vi "Set Value.vi"(7 "TOML string":string, 8 "error in (no error)":errorcluster, 9 "start position":i32, 10 "Value":T3, 11 "Values in":T2[](array[typedef])) -> (0 "error out":errorcluster, 1 "offset past match":i32, 2 "State":T1, 3 "Values out":T2[](array[typedef]))   [LabVIEW 2015, in "JSON.lvlib"]
uses:
  JSON.lvlib
  Value.ctl
  Value Type.ctl
  Context.ctl
  State.ctl
  Object Context.ctl
  Name-Value Pair.ctl
  Array Context.ctl
  <vilib>/regexp/Match Regular Expression.xnode
panel:
  in  "Define":bool=TRUE
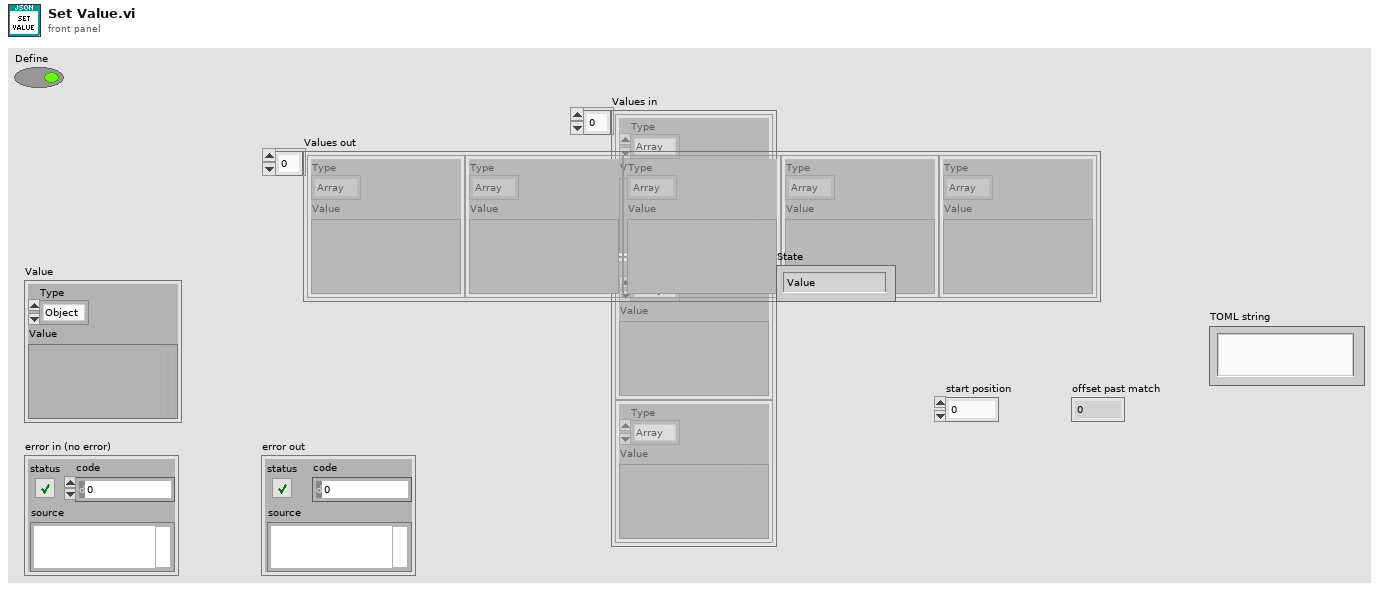
[diagram p1: front panel]
types:
  T1 = typedef "JSON.lvlib/State.ctl" = enum16{"Value", "Object"}
  T2 = typedef "JSON.lvlib/Context.ctl" = cluster{"Type":enum16{"Array", "Object", "Root"}, "Value":variant}
  T3 = typedef "JSON.lvlib/Value.ctl" = cluster{"Type":T4, "Value":variant}
  T4 = typedef "JSON.lvlib/Value Type.ctl" = enum16{"Object", "Array", "String", "Number", "Boolean", "Null"}
  T5 = typedef "JSON.lvlib/Object Context.ctl" = cluster{"Object":T6[], "Key":string}
  T6 = typedef "JSON.lvlib/Name-Value Pair.ctl" = cluster{"Name":string, "Value":T3}
  T7 = typedef "JSON.lvlib/Array Context.ctl" = cluster{"Array":T3[]}
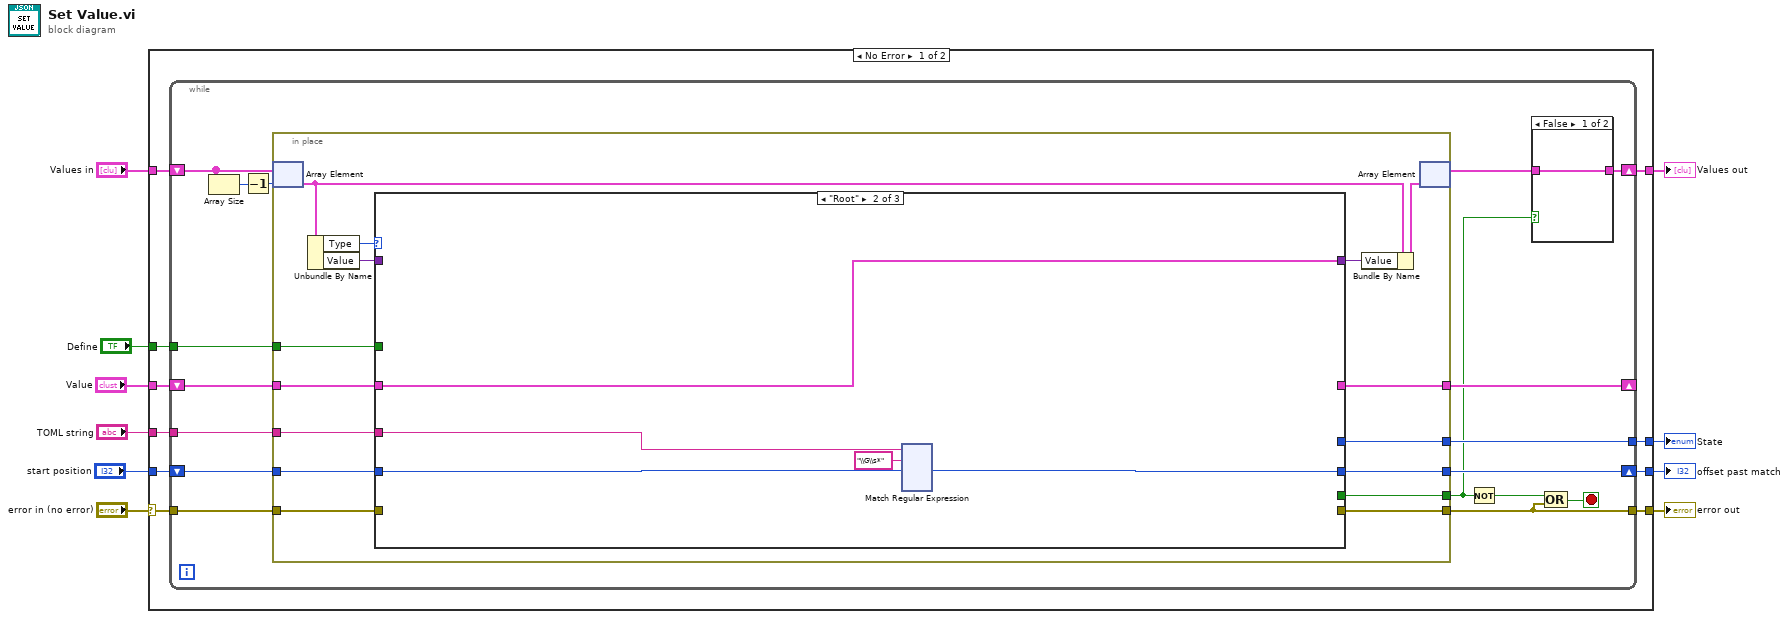
[diagram p0: block diagram]
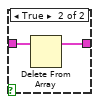
[diagram p2: hidden frame]
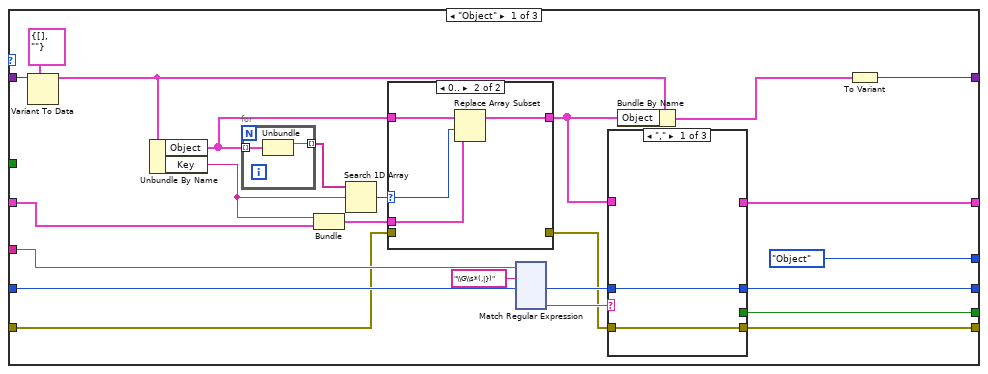
[diagram p3: hidden frame]
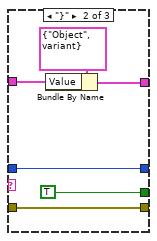
[diagram p4: hidden frame]
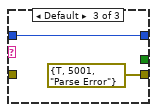
[diagram p5: hidden frame]
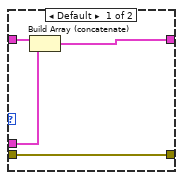
[diagram p6: hidden frame]
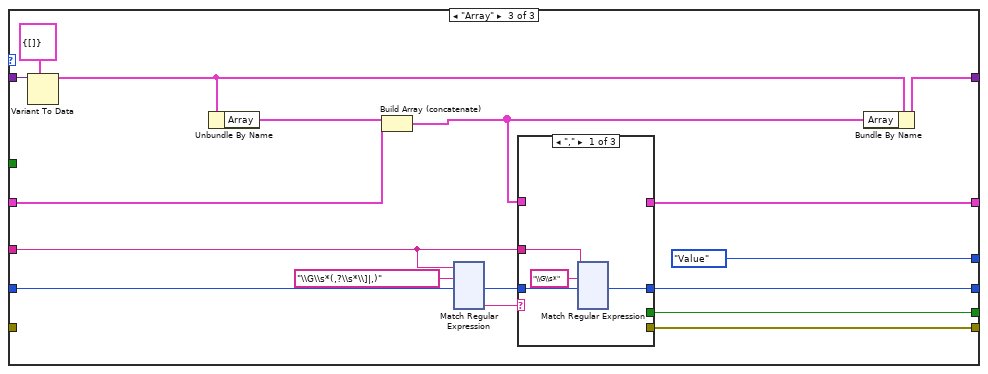
[diagram p7: hidden frame]
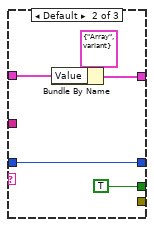
[diagram p8: hidden frame]
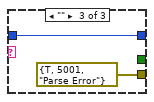
[diagram p9: hidden frame]
diagram:
  n1 = case shown="No Error" "error in (no error)" {
    selector: "error in (no error)" -> [w15 w599]
    tunnel: "Values in" -> [w20 w597]
    tunnel: [w19 w597] -> w9
    tunnel: "Value" -> [w18 _]
    tunnel: [w17 _] -> w7
    tunnel: [w16 w599] -> w6
    tunnel: "start position" -> [w14 w598]
    tunnel: "TOML string" -> [w13 _]
    tunnel: [w12 w598] -> w2
    tunnel: "Define" -> [w11 _]
    frame No Error {
      n2 = while {
        tunnel: [w33] -> w17
        tunnel: w13 -> [w28]
        shift-right: [w26] -> w12
        shift-left: w14 -> [w29]
        tunnel: w15 -> [w32]
        tunnel: [w30] -> w16
        shift-right: [w25] -> _
        shift-left: w18 -> [w34]
        shift-right: [w24] -> w19
        shift-left: w20 -> [w35]
        tunnel: w11 -> [w23]
        stop <- w31 stop-if-true
        n3 = Array Size(array=w35) -> (size(s)=w37:i32)
        n4 = Decrement(x=w37) -> (x-1=w36:i32)
        n5 = in-place {
          in-place-border: w34 -> [w50]
          in-place-border: [w49] -> w33
          in-place-border: [w48] -> w30
          in-place-border: w32 -> [w47]
          in-place-border: [w44] -> w21
          in-place-border: w29 -> [w46]
          in-place-border: w28 -> [w45]
          in-place-border: [w43] -> w25
          in-place-border: [w42] -> w26
          in-place-border: w23 -> [w41]
          n6 = in-place-array #1(w35, w36) -> (w53:T2)
          n7 = Unbundle By Name(w53) -> ("Type"=w55:enum16{"Array", "Object", "Root"}, "Value"=w54:variant)
          n8 = case shown="\"Root\"" w55 {
            tunnel: w54 -> [w79 _ w353]
            tunnel: w50 -> [w73 w220 w342]
            tunnel: [w58 w220 w352] -> w52
            tunnel: [State."Object" ("State") _ State."Value" ("State")] -> w49
            tunnel: [w60 _ w345] -> w48
            tunnel: w47 -> [w57 _ _]
            tunnel: w46 -> [w69 w217 w348]
            tunnel: w45 -> [w68 w218 w344]
            tunnel: [w64 _ w349] -> w44
            tunnel: [w62 _ w346] -> w43
            tunnel: [w61 w216 w347] -> w42
            tunnel: w41 -> [_ _ _]
            frame "Object" {
              n9 = Variant To Data(type=T5 {"Object"=[], "Key"=""} ("Table Context"), Variant=w79) -> (data=w72:T5)  [unwired: 1 in, 1 out]
              n10 = Unbundle By Name(w72) -> ("Object"=w75:T6[], "Key"=w74:string)
              n11 = for {
                tunnel: w75 -> [w215] mode=indexing
                tunnel: [w214] -> w77 mode=indexing
                n12 = Unbundle(w215) -> ("Name"=w214:string)  [unwired: 1 out]
              }
              n13 = Bundle("Key"=w74, "Value"=w73) -> (w71:cluster{"Key":string, "Value":T3})  [unwired: 1 in]
              n14 = Search 1D Array(1D array=w77, element=w74) -> (index of element=w76:i32)  [unwired: 1 in]
              n15 = case shown="0.." w76 {
                selector: w76 -> [_ w212]
                tunnel: w75 -> [w209 w213]
                tunnel: [w208 w210] -> w63
                tunnel: w71 -> [w207 w211]
                tunnel: w57 -> [w206 _]
                tunnel: [w206 _] -> w56
                frame Default {
                  n16 = Build Array (concatenate)(w209, w207) -> (w208:T6[])
                }
                frame 0.. {
                  n17 = Replace Array Subset(array=w213, new element=w211, index=w212) -> (w210:T6[])
                }
              }
              n18 = xnode "Match Regular Expression"("input string"=w68, "regular expression"="\\G\\s*(,|})", "offset (0)"=w69) -> ("offset past match"=w65:i32, "submatch 1"=w66:string)  [unwired: 3 in, 4 out]
              n19 = case shown="\",\"" w66 {
                tunnel: w65 -> [w197 w199 w205]
                tunnel: [_ TRUE _] -> w64
                tunnel: w63 -> [_ w201 _]
                tunnel: [_ w200 _] -> w62
                tunnel: [w197 w199 w205] -> w61
                tunnel: [w196 w198 errorcluster {"status"=TRUE, "code"=5001, "source"="Parse Error"} ("error constant")] -> w60
                tunnel: w56 -> [w196 w198 _]
                frame "," {
                }
                frame "}" {
                  n20 = Bundle By Name(cluster=T3 {"Type"=enum."Object", "Value"=variant} ("Value"), "Value"=w201) -> (w200:T3)
                }
                frame Default {
                }
              }
              n21 = Bundle By Name(cluster=w72, "Object"=w63) -> (w59:T5)
              n22 = To Variant(anything=w59) -> (Variant=w58:variant)
            }
            frame "Root" {
              n23 = xnode "Match Regular Expression"("input string"=w218, "regular expression"="\\G\\s*", "offset (0)"=w217) -> ("offset past match"=w216:i32)  [unwired: 3 in, 5 out]
            }
            frame "Array" {
              n24 = Variant To Data(type=T7 {"Array"=[]} ("Array Context"), Variant=w353) -> (data=w343:T7)  [unwired: 1 in, 1 out]
              n25 = Unbundle By Name(w343) -> ("Array"=w337:T3[])
              n26 = Build Array (concatenate)(w337, w342) -> (w338:T3[])
              n27 = xnode "Match Regular Expression"("input string"=w344, "regular expression"="\\G\\s*(,?\\s*\\]|,)", "offset (0)"=w348) -> ("offset past match"=w339:i32, "submatch 1"=w340:string)  [unwired: 3 in, 4 out]
              n28 = case shown="\",\"" w340 {
                tunnel: w339 -> [w471 w590 w596]
                tunnel: [_ TRUE _] -> w349
                tunnel: w338 -> [_ w592 _]
                tunnel: [_ w591 _] -> w346
                tunnel: [w470 w590 w596] -> w347
                tunnel: [_ _ errorcluster {"status"=TRUE, "code"=5001, "source"="Parse Error"} ("error constant")] -> w345
                tunnel: w344 -> [w472 _ _]
                frame "," {
                  n29 = xnode "Match Regular Expression"("input string"=w472, "regular expression"="\\G\\s*", "offset (0)"=w471) -> ("offset past match"=w470:i32)  [unwired: 3 in, 5 out]
                }
                frame Default {
                  n30 = Bundle By Name(cluster=T3 {"Type"=enum."Array", "Value"=variant} ("Value"), "Value"=w592) -> (w591:T3)
                }
                frame "" {
                }
              }
              n31 = Bundle By Name(cluster=w343, "Array"=w338) -> (w352:T7)
            }
          }
          n32 = Bundle By Name(cluster=w53, "Value"=w52) -> (w51:T2)
          n33 = in-place-array #1(w51) -> (w22:T2[])  [unwired: 1 out]
        }
        n34 = Not(x=w21) -> (.not. x?=w27:bool)
        n35 = case shown="False" w21 {
          tunnel: w22 -> [w38 w40]
          tunnel: [w38 w39] -> w24
          frame False {
          }
          frame True {
            n36 = Delete From Array(array=w40) -> (array with subset deleted=w39:T2[])  [unwired: 2 in, 1 out]
          }
        }
        n37 = Compound Arithmetic op=OR(w27, w30) -> (w31:bool)
      }
    }
    frame Error {
    }
  }
  "error out" <- w6
  "Values out" <- w9
  "State" <- w7
  "offset past match" <- w2
